vi "ReplaceCodes.vi"(8 "Conv String in":string, 11 "String in":string) -> (0 "String out":string, 3 "Conv String out":string)   [LabVIEW 2016]
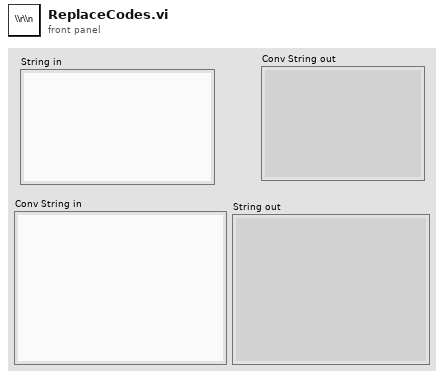
[diagram p1: front panel]
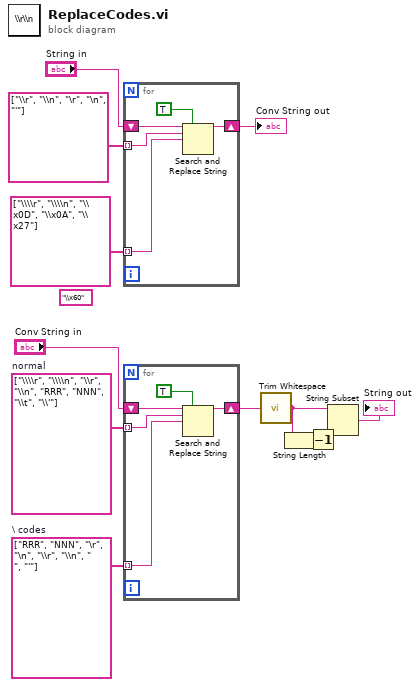
[diagram p0: block diagram]
diagram:
  (unwired) "\\x60"
  w10 = string[] ["\\\\r", "\\\\n", "\\r", "\\n", "RRR", "NNN", "\\t", "\\'"]  # normal
  w9 = string[] ["RRR", "NNN", "\r", "\n", "\\r", "\\n", "     ", "'"]  # \ codes
  n1 = for {
    shift-right: [w15] -> w1
    shift-left: "String in" -> [w17]
    tunnel: string[] ["\\r", "\\n", "\r", "\n", "'"] -> [w14] mode=indexing
    tunnel: string[] ["\\\\r", "\\\\n", "\\x0D", "\\x0A", "\\x27"] -> [w13] mode=indexing
    n2 = Search and Replace String(replace all?=TRUE ("replace all? (F)"), input string=w17, search string=w14, replace string=w13) -> (result string=w15:string)  [unwired: 4 in, 3 out]
  }
  "Conv String out" <- w1
  n3 = for {
    shift-right: [w20] -> w11
    shift-left: "Conv String in" -> [w21]
    tunnel: w10 -> [w19] mode=indexing
    tunnel: w9 -> [w18] mode=indexing
    n4 = Search and Replace String(replace all?=TRUE ("replace all? (F)"), input string=w21, search string=w19, replace string=w18) -> (result string=w20:string)  [unwired: 4 in, 3 out]
  }
  n5 = call <vilib>:"Trim Whitespace.vi"("string"=w11) -> ("trimmed string"=w5:string)  [unwired: 1 in]
  n6 = String Length(string=w5) -> (length=w6:i32)
  n7 = Decrement(x=w6) -> (x-1=w3:i32)
  n8 = String Subset(string=w5, length (rest)=w3) -> (substring=→"String out":string)  [unwired: 1 in]
